vi "MoveTerminalsToBottom.vi"(6 "Error terminals":T1, 7 "Controls [t] / indicators [f]":bool, 8 "error in (no error)":errorcluster, 9 "Case structure contents to move away from":refnum<vi>[](array[refnum]), 11 "VI in":refnum<vi>) -> (0 "error out":errorcluster, 3 "VI ref (dup)":refnum<vi>)   [LabVIEW 2017, in "ErrorStructureDrawer.lvlib"]
doc: "Selects and moves the specified error control or indicator, in order to move it below the specified items (the ones which will end up in the new case structure)."
uses:
  ErrorStructureDrawer.lvlib
  Controls/ErrorTerminals.ctl
  <vilib>/Utility/miscctls.llb/LVDeltaXY32Cluster.ctl
  GetErrorIndicatorVertSpacingBD.vi
  GetErrorControlVertSpacingBD.vi
  GetErrorStructureConstants.vi
  GetErrorStructureInnerWhitespace.vi
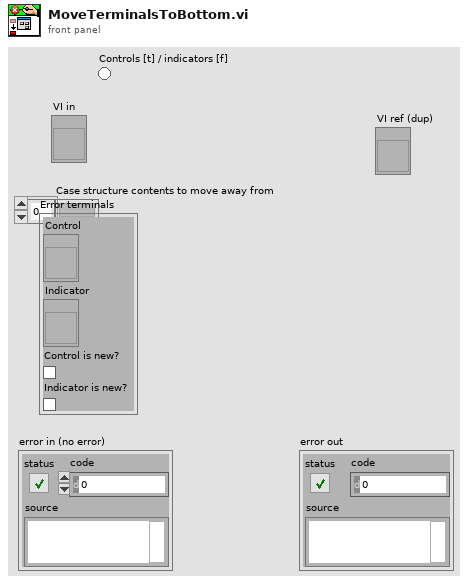
[diagram p1: front panel]
types:
  T1 = typedef "ErrorStructureDrawer.lvlib/ErrorTerminals.ctl" = cluster{"Control":refnum<vi>, "Indicator":refnum<vi>, "Control is new?":bool, "Indicator is new?":bool}
  T2 = typedef "LVDeltaXY32Cluster.ctl" = cluster{"X":i32, "Y":i32}
  T3 = typedef "LVBoundsTypeDef.ctl" = cluster{"Width":u32, "Height":u32}
  T4 = typedef "LVRectTypeDef.ctl" = cluster{"Left":i16, "Top":i16, "Right":i16, "Bottom":i16}
  T5 = typedef "LVPositionTypeDef.ctl" = cluster{"Left":i32, "Top":i32}
  T6 = typedef "ErrorStructureDrawer.lvlib/CaseStructureConstants.ctl" = cluster{"Border thickness":u32, "Case-menu height":u32}
  T7 = typedef "ErrorStructureDrawer.lvlib/CaseStructureInnerWhitespace.ctl" = cluster{"Left":u32, "Right":u32, "Top":u32, "Bottom":u32}
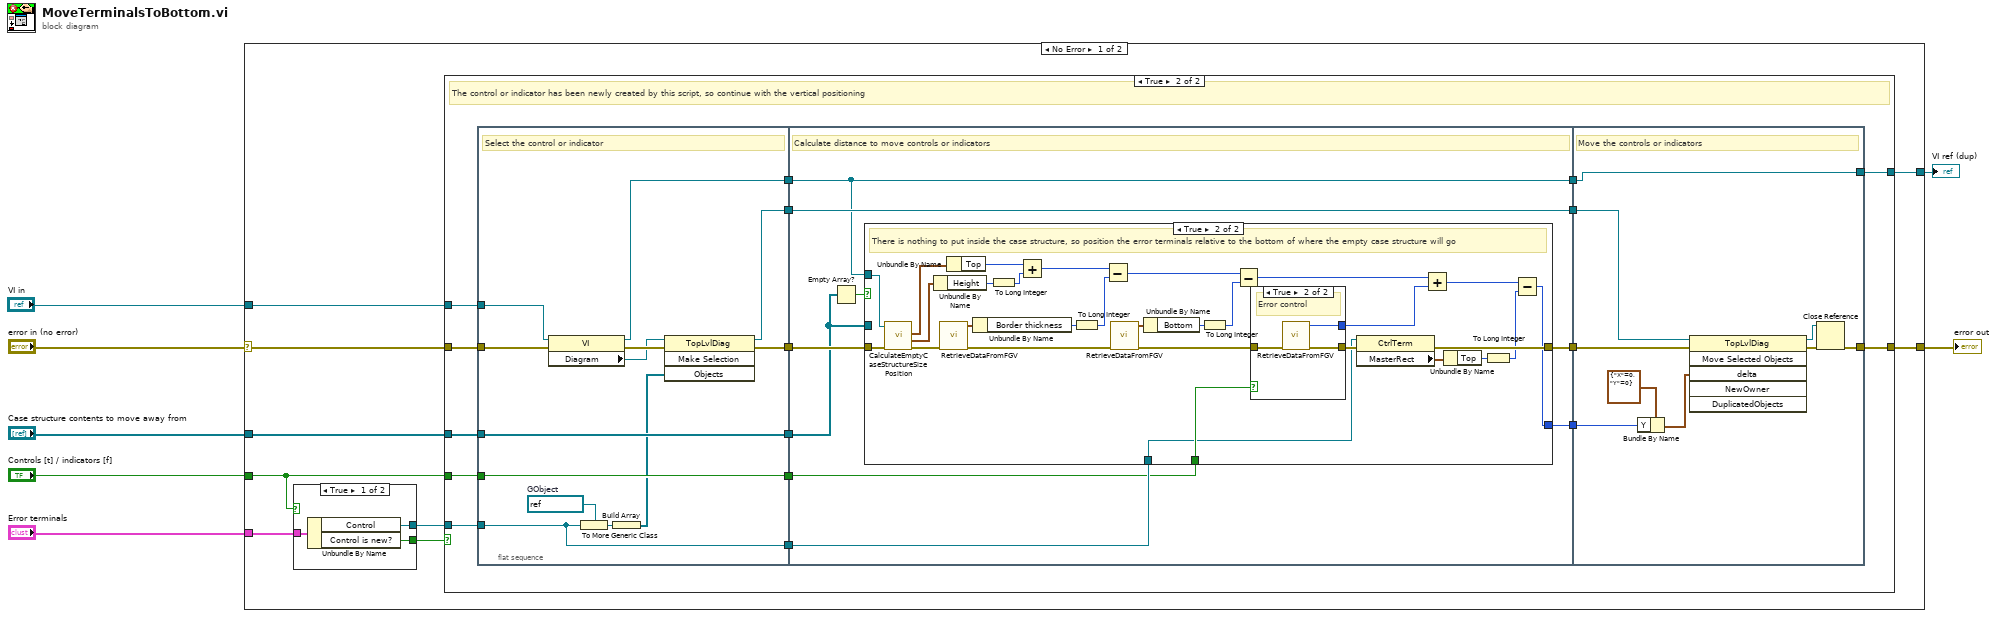
[diagram p0: block diagram]
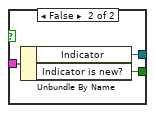
[diagram p2: hidden frame]
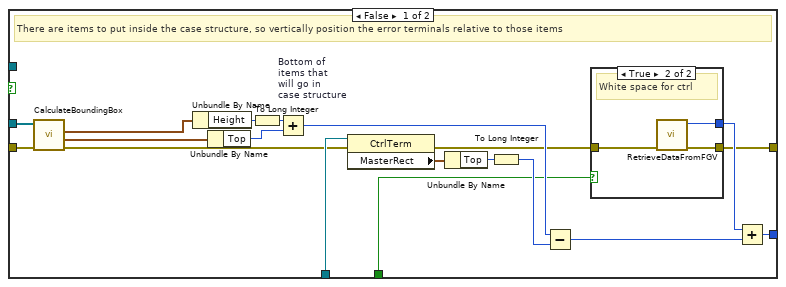
[diagram p4: hidden frame]
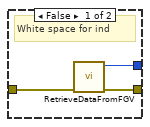
[diagram p5: hidden frame]
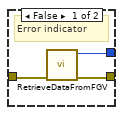
[diagram p6: hidden frame]
diagram:
  n1 = case shown="No Error" "error in (no error)" {
    selector: "error in (no error)" -> [w13 w134]
    tunnel: "Case structure contents to move away from" -> [w16 _]
    tunnel: "Controls [t] / indicators [f]" -> [w9 _]
    tunnel: [w15 w133] -> w1
    tunnel: [w14 w134] -> w5
    tunnel: "Error terminals" -> [w11 _]
    tunnel: "VI in" -> [w12 w133]
    frame No Error {
      n2 = case shown="True" w9 {
        tunnel: w11 -> [w19 w22]
        tunnel: [w18 w21] -> w10
        tunnel: [w17 w20] -> w8
        frame True {
          n3 = Unbundle By Name(w19) -> ("Control"=w18:refnum<vi>, "Control is new?"=w17:bool)
        }
        frame False {
          n4 = Unbundle By Name(w22) -> ("Indicator"=w21:refnum<vi>, "Indicator is new?"=w20:bool)
        }
      }
      n5 = case shown="True" w8 {
        tunnel: w16 -> [_ w31]
        tunnel: w9 -> [_ w26]
        tunnel: [w23 w30] -> w15
        tunnel: [w24 w29] -> w14
        tunnel: w13 -> [w24 w28]
        tunnel: w12 -> [w23 w27]
        tunnel: w10 -> [_ w25]
        frame False {
          # "The control or indicator existing before this script, so don't perform the vertical positioning"
        }
        frame True {
          # "The control or indicator has been newly created by this script, so continue with the vertical positioning"
          n6 = flat-sequence {
            tunnel: w26 -> [w51]
            tunnel: w31 -> [w54]
            tunnel: [w54] -> w41
            tunnel: [w53] -> w40
            tunnel: [w51] -> w39
            tunnel: w28 -> [w47]
            tunnel: [w52] -> w38
            tunnel: [w42] -> w37
            tunnel: w27 -> [w45]
            tunnel: [w43] -> w36
            tunnel: w25 -> [w42]
            tunnel: [w58] -> w35
            tunnel: [w63] -> w34
            tunnel: w41 -> [w56]
            tunnel: w40 -> [w62]
            tunnel: w39 -> [w59]
            tunnel: [w61] -> w33
            tunnel: w38 -> [w61]
            tunnel: w37 -> [w60]
            tunnel: w36 -> [w55]
            tunnel: [w55] -> w32
            tunnel: w35 -> [w129]
            tunnel: w34 -> [w130]
            tunnel: [w124] -> w30
            tunnel: [w125] -> w29
            tunnel: w33 -> [w128]
            tunnel: w32 -> [w124]
            frame #0 {
              w50 = refnum<vi> refnum  # GObject
              # "Select the control or indicator"
              n7 = property class="VI"(reference=w45, error in=w47) -> (reference out=w43:refnum<vi>, error out=w46:errorcluster, "Diagram"=w44:refnum<vi>)
              n8 = To More Generic Class(target class=w50, reference=w42) -> (generic class reference=w49:refnum<vi>)
              n9 = Build Array(w49) -> (w48:refnum<vi>[])
              n10 = invoke class="TopLvlDiag" method="Make Selection"(reference=w44, error in=w46, "Objects"=w48) -> (reference out=w52:refnum<vi>, error out=w53:errorcluster)  [unwired: 1 in, 2 out]
            }
            frame #1 {
              # "Calculate distance to move controls or indicators"
              n11 = Empty Array?(array=w56) -> (empty?=w57:bool)
              n12 = case shown="True" w57 {
                tunnel: [w82 w98] -> w63
                tunnel: w56 -> [w80 _]
                tunnel: w62 -> [w79 w117]
                tunnel: w60 -> [w77 w100]
                tunnel: w59 -> [w66 w105]
                tunnel: [w64 w99] -> w58
                tunnel: w55 -> [_ w104]
                frame False {
                  # "There are items to put inside the case structure, so vertically position the error terminals relative to those items"
                  n13 = call "CalculateBoundingBox.vi"("error in (no error)"=w79, "Items"=w80) -> ("error out"=w67:errorcluster, "Current bounding box position"=w81:cluster{"Left":i32, "Top":i32}, "Size of bounding box for items"=w78:T3)  [unwired: 6 in, 1 out]
                  n14 = Unbundle By Name(w78) -> ("Height"=w74:u32)
                  n15 = Unbundle By Name(w81) -> ("Top"=w75:i32)
                  n16 = To Long Integer(number=w74) -> (32bit integer=w73:i32)
                  n17 = Add "Bottom of\nitems that\nwill go in\ncase structure"(x=w73, y=w75) -> (x+y=w68:i32)
                  n18 = property class="CtrlTerm"(reference=w77, error in=w67) -> (error out=w65:errorcluster, "MasterRect"=w71:T4)  [unwired: 1 out]
                  n19 = Unbundle By Name(w71) -> ("Top"=w70:i16)
                  n20 = To Long Integer(number=w70) -> (32bit integer=w69:i32)
                  n21 = Subtract(x=w68, y=w69) -> (x-y=w76:i32)
                  n22 = case shown="True" w66 {
                    tunnel: [w85 w88] -> w72
                    tunnel: [w84 w87] -> w64
                    tunnel: w65 -> [w83 w86]
                    frame False {
                      # "White space for ind"
                      n23 = call-poly "RetrieveDataFromFGV.vi"("error in (no error)"=w83) -> ("error out"=w84:errorcluster, "Error indicator vertical spacing from existing BD items"=w85:i32)  [unwired: 9 in]
                    }
                    frame True {
                      # "White space for ctrl"
                      n24 = call-poly "RetrieveDataFromFGV.vi"("error in (no error)"=w86) -> ("error out"=w87:errorcluster, "Error control vertical spacing from existing BD items"=w88:i32)  [unwired: 9 in]
                    }
                  }
                  n25 = Add(x=w72, y=w76) -> (x+y=w82:i32)
                }
                frame True {
                  # "There is nothing to put inside the case structure, so position the error terminals relative to the bottom of where the empty case structure will go"
                  n26 = call "CalculateEmptyCaseStructureSizePosition.vi"("error in (no error)"=w117, "VI ref in"=w104) -> ("error out"=w106:errorcluster, "Case structure frame size"=w115:T3, "Case structure position"=w116:T5)  [unwired: 6 in, 1 out]
                  n27 = Unbundle By Name(w115) -> ("Height"=w110:u32)
                  n28 = call-poly "RetrieveDataFromFGV.vi"("error in (no error)"=w106) -> ("error out"=w90:errorcluster, "Case structure constants"=w112:T6)  [unwired: 9 in]
                  n29 = Unbundle By Name(w116) -> ("Top"=w114:i32)
                  n30 = Unbundle By Name(w112) -> ("Border thickness"=w108:u32)
                  n31 = To Long Integer(number=w110) -> (32bit integer=w109:i32)
                  n32 = Add(x=w114, y=w109) -> (x+y=w113:i32)
                  n33 = To Long Integer(number=w108) -> (32bit integer=w107:i32)
                  n34 = Subtract(x=w113, y=w107) -> (x-y=w111:i32)
                  n35 = call-poly "RetrieveDataFromFGV.vi"("error in (no error)"=w90) -> ("error out"=w89:errorcluster, "Case structure inner whitespace (px)"=w96:T7)  [unwired: 9 in]
                  n36 = Unbundle By Name(w96) -> ("Bottom"=w92:u32)
                  n37 = To Long Integer(number=w92) -> (32bit integer=w91:i32)
                  n38 = Subtract(x=w111, y=w91) -> (x-y=w95:i32)
                  n39 = case shown="True" w105 {
                    tunnel: [w118 w123] -> w93
                    tunnel: [w119 w122] -> w101
                    tunnel: w89 -> [w120 w121]
                    frame False {
                      # "Error indicator"
                      n40 = call-poly "RetrieveDataFromFGV.vi"("error in (no error)"=w120) -> ("error out"=w119:errorcluster, "Error indicator vertical spacing from existing BD items"=w118:i32)  [unwired: 9 in]
                    }
                    frame True {
                      # "Error control"
                      n41 = call-poly "RetrieveDataFromFGV.vi"("error in (no error)"=w121) -> ("error out"=w122:errorcluster, "Error control vertical spacing from existing BD items"=w123:i32)  [unwired: 9 in]
                    }
                  }
                  n42 = property class="CtrlTerm"(reference=w100, error in=w101) -> (error out=w99:errorcluster, "MasterRect"=w102:T4)  [unwired: 1 out]
                  n43 = Add(x=w95, y=w93) -> (x+y=w94:i32)
                  n44 = Unbundle By Name(w102) -> ("Top"=w103:i16)
                  n45 = To Long Integer(number=w103) -> (32bit integer=w97:i32)
                  n46 = Subtract(x=w94, y=w97) -> (x-y=w98:i32)
                }
              }
            }
            frame #2 {
              # "Move the controls or indicators"
              n47 = Bundle By Name(cluster=T2 {"X"=0, "Y"=0} ("X/Y Delta"), "Y"=w130) -> (w132:T2)
              n48 = invoke class="TopLvlDiag" method="Move Selected Objects"(reference=w128, error in=w129, "delta"=w132) -> (reference out=w126:refnum<vi>, error out=w127:errorcluster)  [unwired: 3 in, 4 out]
              n49 = Close Reference(reference=w126, error in (no error)=w127) -> (error out=w125:errorcluster)
            }
          }
        }
      }
    }
    frame Error {
    }
  }
  "error out" <- w5
  "VI ref (dup)" <- w1
